vi "Chronos Update Limit Plots.vi"(8 "error in (no error)":errorcluster, 10 "End Time":dbl, 11 "Limits":T1) -> (0 "error out":errorcluster, 3 "Limits out":T1)   [LabVIEW 2021]
uses:
  Chronos cluster Map Limit Plots.ctl
  typedefs/Chronos cluster Plot Data and Limits.ctl
  Viewer/cluster CC Channel from TDMS.ctl
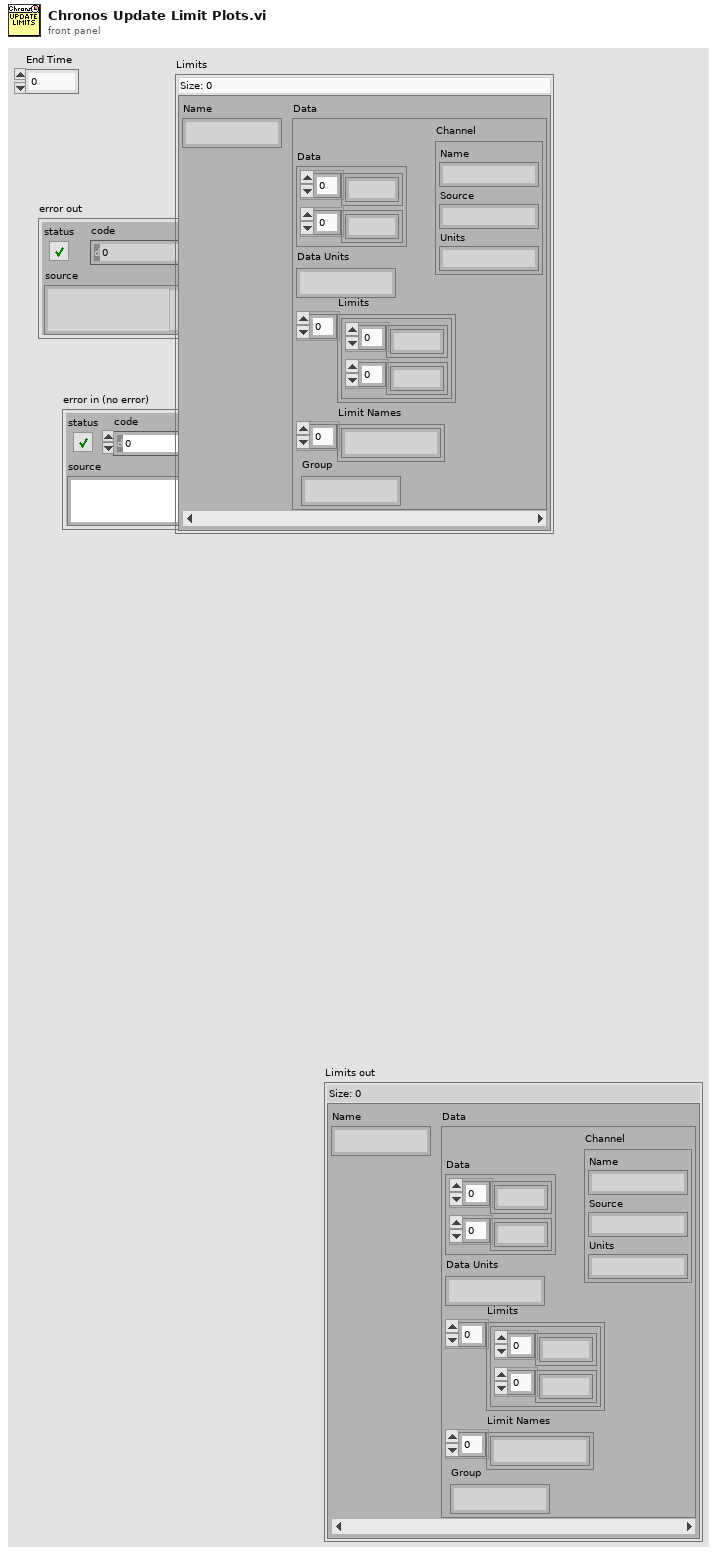
[diagram p1: front panel]
types:
  T1 = typedef "Chronos cluster Map Limit Plots.ctl" = map{string, T2}
  T2 = typedef "Chronos cluster Plot Data and Limits.ctl" = cluster{"Data":cluster{dbl[], dbl[]}, "Data Units":string, "Limits":cluster{dbl[], dbl[]}[], "Limit Names":string[], "Channel":T3, "Group":string}
  T3 = typedef "cluster CC Channel from TDMS.ctl" = cluster{"Name":string, "Source":string, "Units":string}
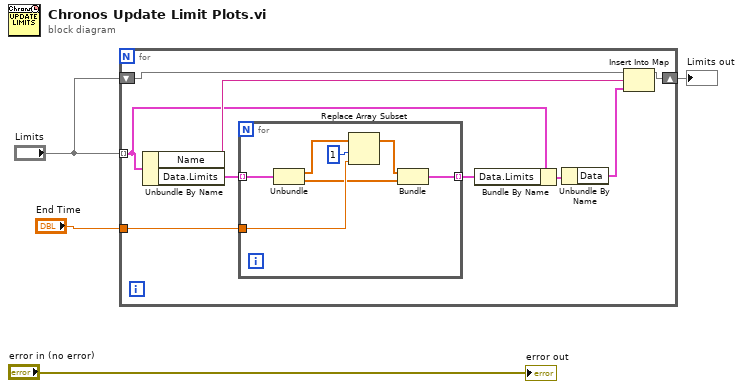
[diagram p0: block diagram]
diagram:
  n1 = for {
    tunnel: "Limits" -> [w9] mode=indexing
    tunnel: "End Time" -> [w12]
    shift-right: [w5] -> w1
    shift-left: "Limits" -> [w11]
    n2 = Unbundle By Name(w9) -> ("Name"=w10:string, "Data.Limits"=w13:cluster{dbl[], dbl[]}[])
    n3 = for {
      tunnel: w13 -> [w18] mode=indexing
      tunnel: w12 -> [w19]
      tunnel: [w14] -> w8 mode=indexing
      n4 = Unbundle(w18) -> (w17:dbl[], w15:dbl[])
      n5 = Replace Array Subset(array=w17, new element=w19, index=1) -> (w16:dbl[])
      n6 = Bundle(w16, w15) -> (w14:cluster{dbl[], dbl[]})  [unwired: 1 in]
    }
    n7 = Bundle By Name(cluster=w9, "Data.Limits"=w8) -> (w7:cluster{"Name":string, "Data":T2})
    n8 = Unbundle By Name(w7) -> ("Data"=w6:T2)
    n9 = Insert Into Map(map in=w11, key=w10, value=w6) -> (map out=w5:T1)  [unwired: 2 out]
  }
  "Limits out" <- w1
  "error out" <- "error in (no error)"
